vi "_init_vartree.vi"(8 "error in (no error)":errorcluster, 10 "config?":bool, 11 "appended path":path) -> (0 "error out":errorcluster, 2 "vartree":T1 {"perms" format="0x%02x"; "vars"."data" format="0x%08x"})   [LabVIEW 2014]
doc: "This VI populates both the system flat variable tree returned in <B>vartree</B> and the system hierarchical variable tree kept inside the 'ahc_utils' dynamic link library. The VI uses the contents of the file 'sysvarcfg.xml' to get the variable definitions.\n\nThe VI handles error status with clusters <B>error_in</B> and <B>error_out</B>.\n\nThe VI must be informed with the configured operation mode in <B>config?</B> in order to add to the list and tree the appropriate variables and permissions."
uses:
  typedefs/vartree_t.ctl
  typedefs/var_t.ctl
  typedefs/val_type_t.ctl
  <vilib>/Utility/xml.llb/Read From XML File(string).vi
  CompactRio/libahcutils.dll
panel:
  out "c":u32
  out "lv":u32
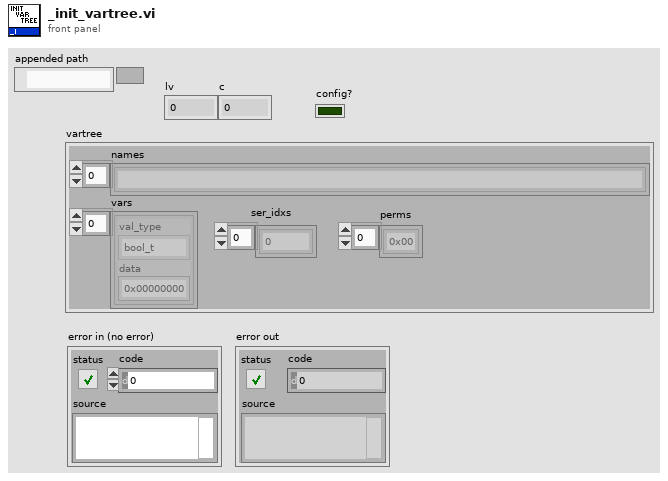
[diagram p1: front panel]
types:
  T1 = typedef "vartree_t.ctl" = cluster{"names":string[], "vars":T2[], "ser_idxs":i32[], "perms":u8[]}
  T2 = typedef "var_t.ctl" = cluster{"data":u32, "val_type":T3}
  T3 = typedef "val_type_t.ctl" = enum16{"bool_t", "i32_t", "u32_t", "f32_t"}
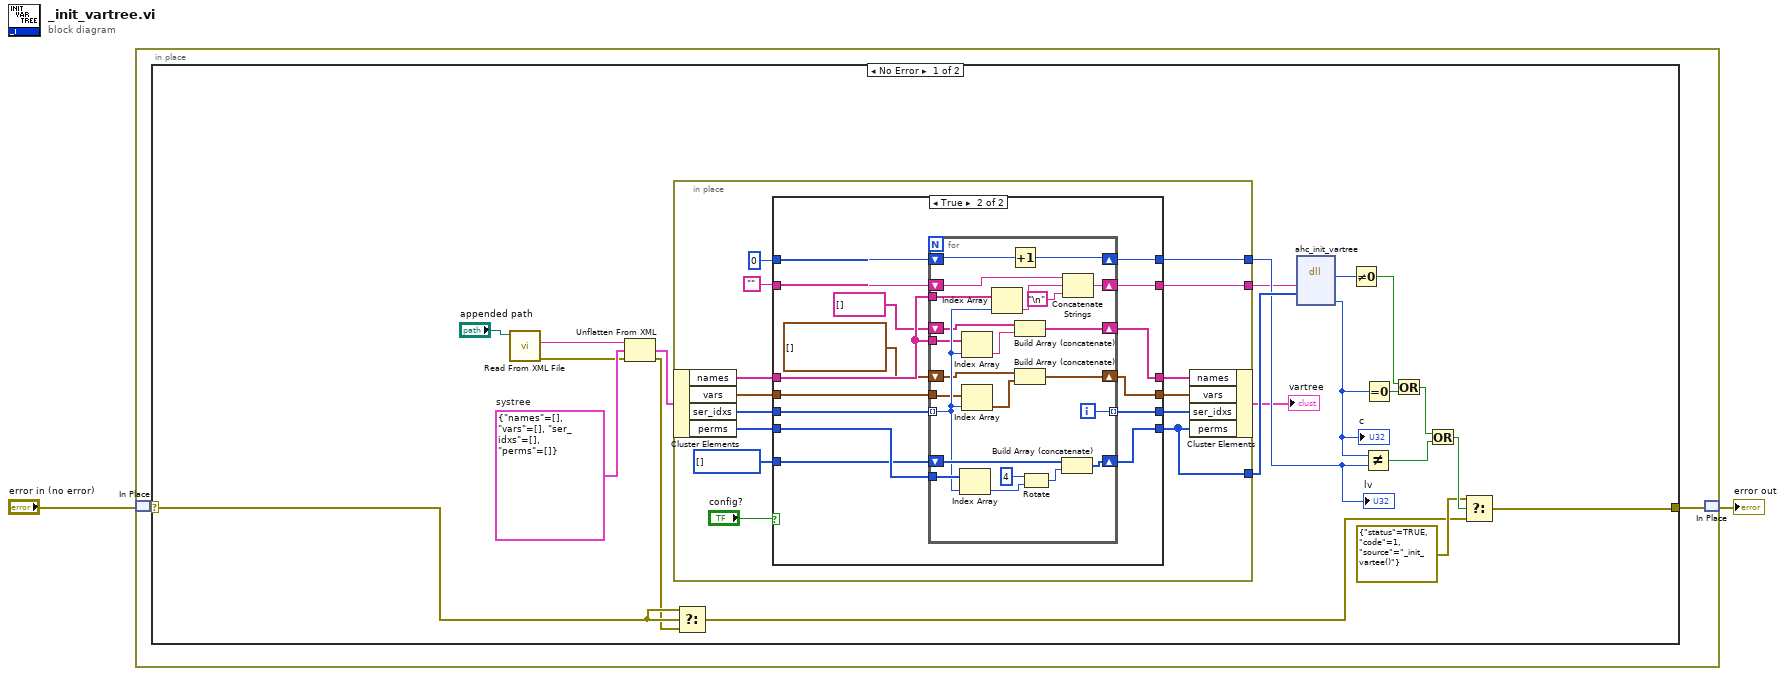
[diagram p0: block diagram]
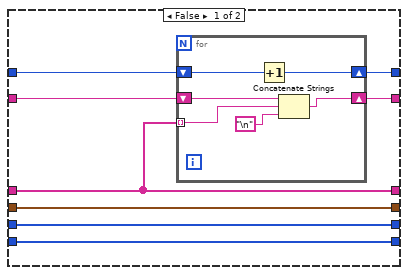
[diagram p2: hidden frame]
diagram:
  n1 = in-place {
    n2 = in-place-match #1("error in (no error)") -> (w4:errorcluster)
    n3 = case shown="No Error" w4 {
      selector: w4 -> [w11 w92]
      tunnel: [w22 w92] -> w3
      frame No Error {
        w24 = T1 {"names"=[], "vars"=[], "ser_idxs"=[], "perms"=[]}  # systree
        n4 = call-poly <vilib>:"Read From XML File.vi"("XML File Path"="appended path") -> ("error out"=w12:errorcluster, "XML Elements"=w25:string)  [unwired: 8 in, 1 out]
        n5 = Unflatten From XML(xml string=w25, type=w24, error in (no error)=w12) -> (value=w14:T1, error out=w10:errorcluster)
        n6 = in-place {
          in-place-border: [w34] -> w15
          in-place-border: [w29] -> w16
          in-place-border: [w28] -> w17
          n7 = in-place-cluster #2(w14) -> ("names"=w33:string[], "vars"=w31:T2[], "ser_idxs"=w35:i32[], "perms"=w37:u8[])
          n8 = case shown="True" "config?" {
            tunnel: "" -> [w47 w67]
            tunnel: w33 -> [w40 w59]
            tunnel: [w46 w64] -> w34
            tunnel: u32 0 ("lv") -> [w45 w66]
            tunnel: [w44 w65] -> w29
            tunnel: w37 -> [w42 w63]
            tunnel: u8[] [] -> [_ w62]
            tunnel: [w42 w61] -> w28
            tunnel: w35 -> [w43 w68]
            tunnel: [w43 w60] -> w26
            tunnel: [w41 w57] -> w32
            tunnel: w31 -> [w41 w58]
            tunnel: [w40 w56] -> w30
            frame False {
              n9 = for {
                tunnel: w40 -> [w48] mode=indexing
                shift-right: [w53] -> w46
                shift-left: w47 -> [w49]
                shift-right: [w51] -> w44
                shift-left: w45 -> [w52]
                n10 = Increment(x=w52) -> (x+1=w51:u32)
                n11 = Concatenate Strings(w49, w48, "\n") -> (w53:string)
              }
            }
            frame True {
              n12 = for {
                tunnel: w68 -> [w77] mode=indexing
                tunnel: w59 -> [w91]
                shift-right: [w89] -> w64
                shift-left: w67 -> [w88]
                shift-right: [w86] -> w65
                shift-left: w66 -> [w87]
                tunnel: w63 -> [w85]
                shift-right: [w83] -> w61
                shift-left: w62 -> [w84]
                tunnel: [w79] -> w60 mode=indexing
                tunnel: w59 -> [w76]
                tunnel: w58 -> [w75]
                shift-right: [w73] -> w56
                shift-left: string[] [] -> [w69]
                shift-right: [w71] -> w57
                shift-left: T2[] [] -> [w70]
                i -> [w79]
                n13 = Index Array(array=w85, index=w77) -> (element=w81:u8)
                n14 = Index Array(array=w76, index=w77) -> (element=w74:string)
                n15 = Index Array(array=w75, index=w77) -> (element=w72:T2)
                n16 = Index Array(array=w91, index=w77) -> (element=w78:string)
                n17 = Increment(x=w87) -> (x+1=w86:u32)
                n18 = Build Array (concatenate)(w69, w74) -> (w73:string[])
                n19 = Build Array (concatenate)(w70, w72) -> (w71:T2[])
                n20 = Rotate(1:w81, 2:i16 4 ("y")) -> (0:w80:u8)
                n21 = Build Array (concatenate)(w84, w80) -> (w83:u8[])
                n22 = Concatenate Strings(w88, w78, "\n") -> (w89:string)
              }
            }
          }
          n23 = in-place-cluster #2("names"=w30, "vars"=w32, "ser_idxs"=w26, "perms"=w28) -> (→"vartree":T1)
        }
        "lv" <- w16
        n24 = Select(t=w11, s=w11, f=w10) -> (s? t:f=w9:errorcluster)
        n25 = dll-call lib="F:/Owncloud/MJR-AHC_System/ScadaHMI/Development/DriverApp/DriverCommApp/DriverComm/XWave/Development/CompactRio/libahcutils.dll" fn="ahc_init_vartree"("vartreedef"=w15, "perms"=w17) -> ("return type"=w6:i32, "nvars"=w20:u32)  [unwired: 6 in, 2 out]
        "c" <- w20
        n26 = Not Equal To 0?(x=w6) -> (x != 0?=w7:bool)
        n27 = Not Equal?(x=w20, y=w16) -> (x != y?=w8:bool)
        n28 = Equal To 0?(x=w20) -> (x = 0?=w19:bool)
        n29 = Or(x=w7, y=w19) -> (x .or. y?=w18:bool)
        n30 = Or(x=w18, y=w8) -> (x .or. y?=w23:bool)
        n31 = Select(t=errorcluster {"status"=TRUE, "code"=1, "source"="_init_vartee()"}, s=w23, f=w9) -> (s? t:f=w22:errorcluster)
      }
      frame Error {
      }
    }
    n32 = in-place-match #1(w3) -> (→"error out":errorcluster)
  }
